vi "Read Frequency.vi"(8 "error in (no error)":errorcluster, 11 "Composite Waveform in":refnum<class "Composite Waveform.lvclass">) -> (0 "error out":errorcluster, 2 "Frequency":dbl, 3 "Composite Waveform out":refnum<class "Composite Waveform.lvclass">)   [LabVIEW 2020, in "Composite Waveform.lvclass"]
uses:
  Composite Waveform.lvclass
  Analog Waveform/Analog Waveform.lvclass
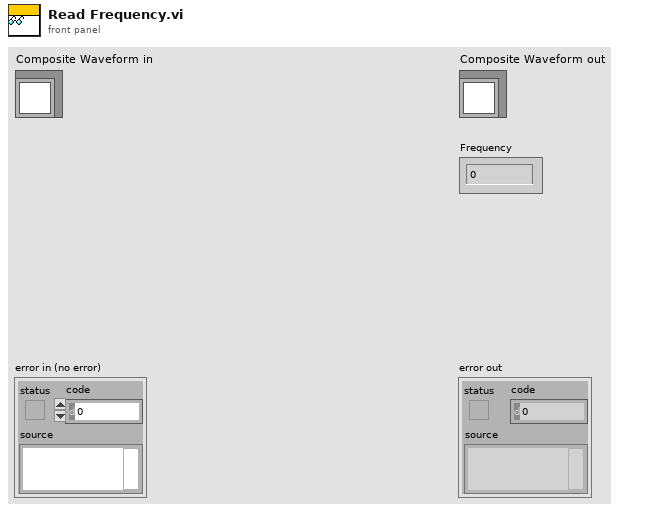
[diagram p1: front panel]
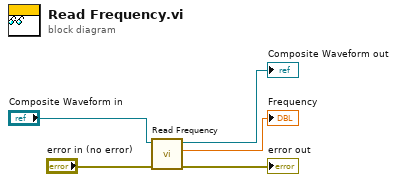
[diagram p0: block diagram]
diagram:
  n1 = call-parent "Read Frequency.vi"("error in (no error)"="error in (no error)", "Analog Waveform in"="Composite Waveform in") -> ("error out"=→"error out":errorcluster, "Frequency"=→"Frequency":dbl, "Analog Waveform out"=→"Composite Waveform out":refnum<class "Composite Waveform.lvclass">)  [unwired: 7 in]
